vi "install_SW_on Target[Save in V2010].vi"() -> ()   [LabVIEW 2010]
uses:
  <vilib>/nisyscfg/nisyscfg.lvlib
  <vilib>/nisyscfg/Initialize (Control).vi
  <vilib>/nisyscfg/Install All 1.0.vi
  <vilib>/nisyscfg/Close (System).vi
  <vilib>/nisyscfg/Get Installed Components 1.0.vi
  <vilib>/nisyscfg/Software.ctl
panel:
  out "Installed Software":T1[](array[typedef])
  out "Installer Beeing installed":i32
  out "Installer present":i32
  out "Software Components":T1[](array[typedef]) caption="SW Summary"
  in  "Target (localhost)":refnum<k21>="localhost"
  out "error out":errorcluster
  in  "error in (no error)":errorcluster
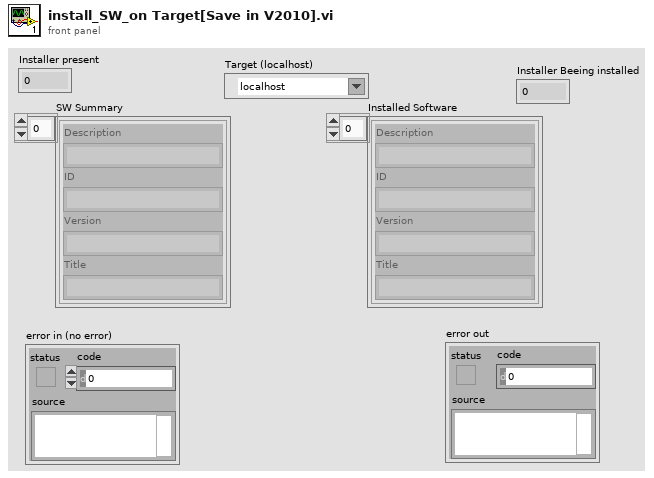
[diagram p1: front panel]
types:
  T1 = typedef "nisyscfg.lvlib/Software.ctl" = cluster{"Description":string, "ID":string, "Version":string, "Title":string}
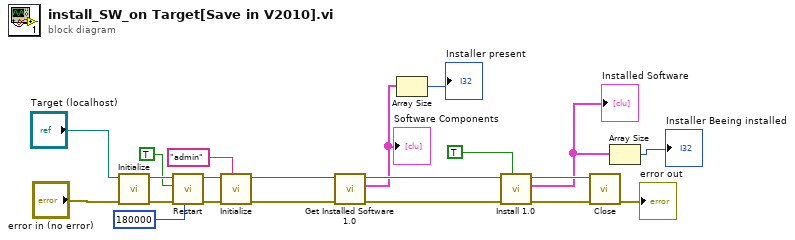
[diagram p0: block diagram]
diagram:
  n1 = call-poly <vilib>:"Initialize.vi"("error in (no error)"="error in (no error)", "Target (localhost)"="Target (localhost)") -> ("error out"=w21:errorcluster, "Session out"=w20:refnum<k21>)  [unwired: 7 in, 1 out]
  n2 = call <vilib>:"Restart.vi"("Timeout (180,000 ms)"=u32 180000, "error in (no error)"=w21, "Install Mode (F)"=TRUE, "Session in"=w20) -> ("error out"=w18:errorcluster, "Session out"=w17:refnum<k21>)  [unwired: 5 in, 1 out]
  n3 = call-poly <vilib>:"Initialize.vi"("User Name"="admin", "error in (no error)"=w18, "Target (localhost)"=w17) -> ("error out"=w7:errorcluster, "Session out"=w8:refnum<k21>)  [unwired: 6 in, 1 out]
  n4 = call-poly <vilib>:"Get Installed Software 1.0.vi"("error in (no error)"=w7, "Session in"=w8) -> ("error out"=w6:errorcluster, "Software Components"=w4:T1[], "Session out"=w5:refnum<k21>)  [unwired: 7 in]
  "Software Components" <- w4
  n5 = Array Size(array=w4) -> (size(s)=→"Installer present":i32)
  n6 = call-poly <vilib>:"Install 1.0.vi"("Restart Automatically (T)"=TRUE, "error in (no error)"=w6, "Session in"=w5) -> ("error out"=w10:errorcluster, "Installed Software"=w2:T1[], "Session out"=w11:refnum<k21>)  [unwired: 5 in, 1 out]
  "Installed Software" <- w2
  n7 = call-poly <vilib>:"Close.vi"("error in (no error)"=w10, "Session in"=w11) -> ("error out"=→"error out":errorcluster)  [unwired: 9 in]
  n8 = Array Size(array=w2) -> (size(s)=→"Installer Beeing installed":i32)
